vi "set_user.vi"(7 "set reference disabled? (F)":bool, 8 "error in (no error)":errorcluster, 9 "ref username in":refnum<vi>, 10 "username in":string) -> (0 "error out":errorcluster)   [LabVIEW 2010]
doc: "Wire a username or a reference of a combo box"
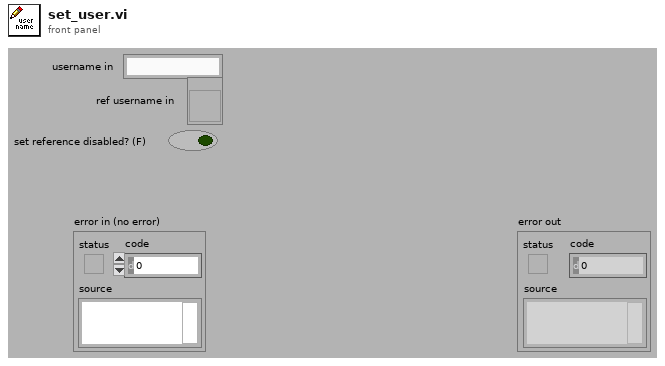
[diagram p1: front panel]
types:
  T1 = enum8{"Enabled", "Disabled", "Disabled and Grayed Out"}
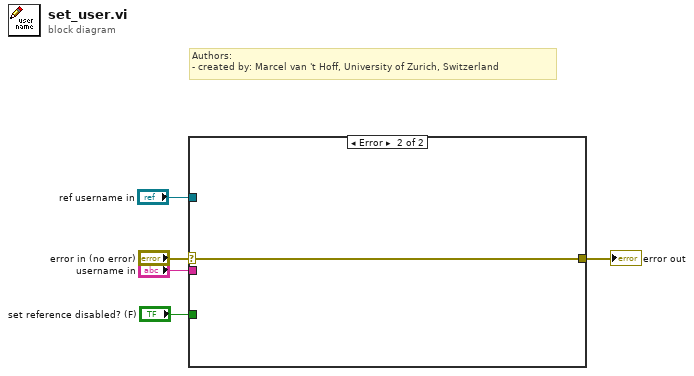
[diagram p0: block diagram]
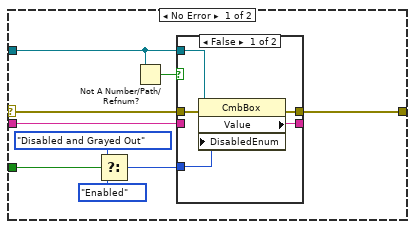
[diagram p2: hidden frame]
diagram:
  # "Authors: \n- created by: Marcel van 't Hoff, University of Zurich, Switzerland"
  n1 = case shown="Error" "error in (no error)" {
    selector: "error in (no error)" -> [w12 w22]
    tunnel: [w11 w22] -> w4
    tunnel: "username in" -> [w13 _]
    tunnel: "ref username in" -> [w14 _]
    tunnel: "set reference disabled? (F)" -> [w9 _]
    frame No Error {
      n2 = Select(t=T1."Disabled and Grayed Out" ("Disabled"), s=w9, f=T1."Enabled" ("Disabled")) -> (s? t:f=w6:T1)
      n3 = Not A Number/Path/Refnum?(number/path/refnum=w14) -> (NaN/Path/Refnum?=w10:bool)
      n4 = case shown="False" w10 {
        tunnel: w14 -> [w19 _]
        tunnel: w12 -> [w18 w20]
        tunnel: [w17 w21] -> _
        tunnel: w13 -> [_ w21]
        tunnel: [w16 w20] -> w11
        tunnel: w6 -> [w15 _]
        frame False {
          n5 = property class="CmbBox"(reference=w19, error in=w18, "DisabledEnum"=w15) -> (error out=w16:errorcluster, "Value"=w17:string)  [unwired: 1 out]
        }
        frame True {
        }
      }
    }
    frame Error {
    }
  }
  "error out" <- w4
